vi "ResMgr-Request TagMap.vi"(6 "Timeout In ms (5000 ms)":i32=5000, 7 "WatchDogQ":refnum<queue>, 8 "Error In":errorcluster caption="error in (no error)") -> (0 "error out":errorcluster, 3 "Data Value Reference":refnum<data-value>)   [LabVIEW 2017, in "Communicable State Machine.lvlib"]
uses:
  Communicable State Machine.lvlib
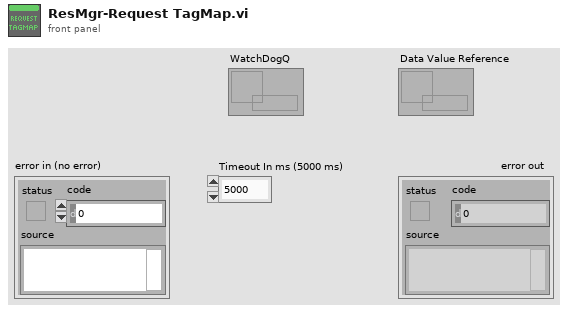
[diagram p1: front panel]
types:
  T1 = cluster{"ResType":string, "RespQ":refnum<queue>, "Parameter":string, "WatchDogQ":refnum<queue>}
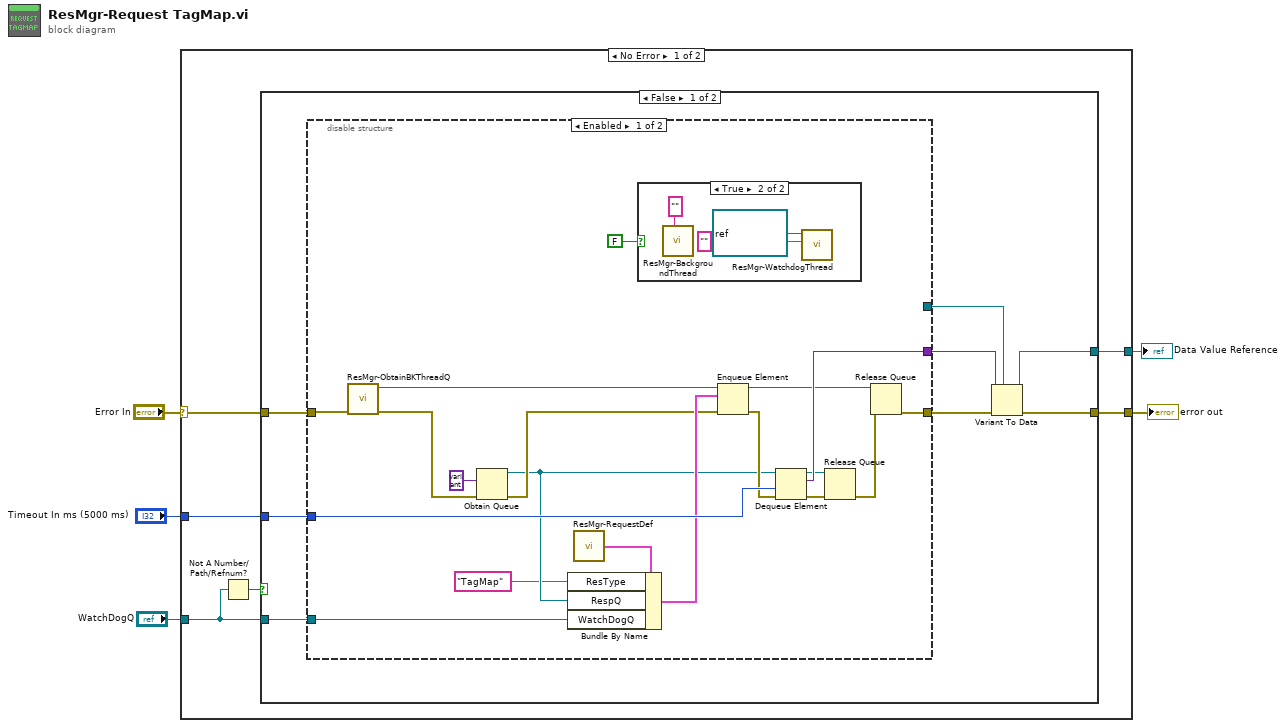
[diagram p0: block diagram]
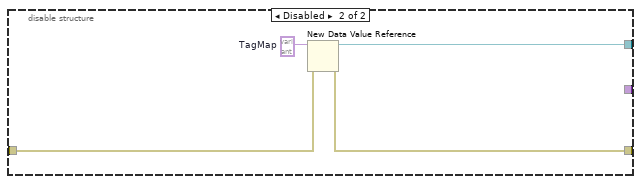
[diagram p3: hidden frame]
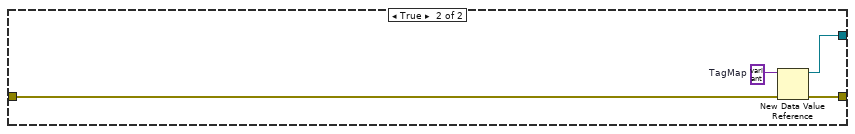
[diagram p4: hidden frame]
diagram:
  n1 = case shown="No Error" "Error In" {
    selector: "Error In" -> [w10 w50]
    tunnel: [w9 w50] -> w5
    tunnel: [w8 _] -> w1
    tunnel: "Timeout In ms (5000 ms)" -> [w11 _]
    tunnel: "WatchDogQ" -> [w7 _]
    frame No Error {
      n2 = Not A Number/Path/Refnum?(number/path/refnum=w7) -> (NaN/Path/Refnum?=w6:bool)
      n3 = case shown="False" w6 {
        tunnel: w11 -> [w18 _]
        tunnel: w10 -> [w17 w46]
        tunnel: w7 -> [w16 _]
        tunnel: [w15 w48] -> w9
        tunnel: [w12 w47] -> w8
        frame False {
          n4 = disable-structure shown="Enabled" {
            disable-tunnel: [w38 w42] -> w19
            disable-tunnel: w18 -> [w37 _]
            disable-tunnel: [w36 _] -> w14
            disable-tunnel: w17 -> [w21 w43]
            disable-tunnel: w16 -> [w25 _]
            disable-tunnel: [_ w44] -> w13
            frame Enabled {
              n5 = call "ResMgr-ObtainBKThreadQ.vi"("error in (no error)"=w21) -> ("error out"=w22:errorcluster, "ObtainBKThreadQ"=w23:refnum<queue>)  [unwired: 9 in]
              n6 = Obtain Queue(element data type=variant, error in (no error)=w22) -> (queue out=w26:refnum<queue>, error out=w34:errorcluster)  [unwired: 3 in, 1 out]
              n7 = call "ResMgr-RequestDef.vi"() -> ("ResMgr-RequestDef.ctl"=w20:T1)  [unwired: 2 in]
              n8 = Bundle By Name(cluster=w20, "ResType"="TagMap", "RespQ"=w26, "WatchDogQ"=w25) -> (w35:T1)
              n9 = case shown="True" FALSE {
                frame False {
                }
                frame True {
                  n10 = call "ResMgr-BackgroundThread.vi"("Name (Unnamed)"="" ("name (unnamed)")) -> ()  [unwired: 11 in]
                  n11 = call "ResMgr-WatchdogThread.vi"("From Who"="", "WatchDogQ"=refnum<queue> refnum) -> ()  [unwired: 10 in]
                }
              }
              n12 = Enqueue Element(queue=w23, element=w35, error in (no error)=w34) -> (queue out=w30:refnum<queue>, error out=w33:errorcluster)  [unwired: 1 in, 1 out]
              n13 = Dequeue Element(queue=w26, timeout in ms (-1)=w37, error in (no error)=w33) -> (queue out=w31:refnum<queue>, element=w36:variant, error out=w32:errorcluster)  [unwired: 1 out]
              n14 = Release Queue(queue=w31, error in (no error)=w32) -> (error out=w29:errorcluster)  [unwired: 1 in, 2 out]
              n15 = Release Queue(queue=w30, error in (no error)=w29) -> (error out=w38:errorcluster)  [unwired: 1 in, 2 out]
            }
            frame Disabled {
              w45 = variant  # TagMap
              n16 = New Data Value Reference(data value=w45, error in=w43) -> (data value reference=w44:refnum<data-value>, error out=w42:errorcluster)
            }
          }
          n17 = Variant To Data(error in=w19, type=w13, Variant=w14) -> (data=w12:refnum<data-value>, error out=w15:errorcluster)
        }
        frame True {
          w49 = variant  # TagMap
          n18 = New Data Value Reference(data value=w49, error in=w46) -> (data value reference=w47:refnum<data-value>, error out=w48:errorcluster)
        }
      }
    }
    frame Error {
    }
  }
  "error out" <- w5
  "Data Value Reference" <- w1
